vi "UDP 쓰기.vi"() -> ()   [LabVIEW 2014]
panel:
  in  "이름":string
  out "주소":u32
  in  "데이터 입력":string
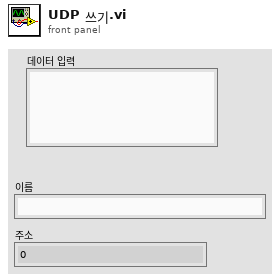
[diagram p1: front panel]
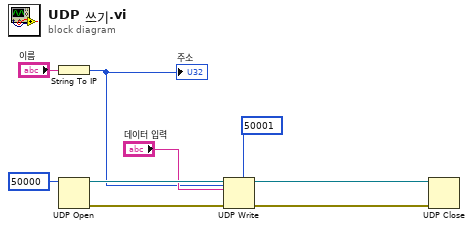
[diagram p0: block diagram]
diagram:
  n1 = String To IP(1:"이름") -> (0:w1:u32)
  "주소" <- w1
  n2 = UDP Open(11:u16 50000 ("포트")) -> (port=w9:refnum<k16>, 0:w7:errorcluster)  [unwired: 4 in, 1 out]
  n3 = UDP Write(address=w1, port or service name=u16 50001 ("포트 또는 서비스 이름"), connection ID=w9, data in="데이터 입력", 8:w7) -> (error out=w6:errorcluster, 3:w8:refnum<k16>)  [unwired: 1 in]
  n4 = UDP Close(connection ID=w8, 8:w6) -> ()  [unwired: 2 out]
